vi "rdb_json_error.vi"(7 "message":string, 8 "error in (no error)":errorcluster, 10 "offset (0)":i32, 11 "json":string) -> (0 "error out":errorcluster)   [LabVIEW 2017]
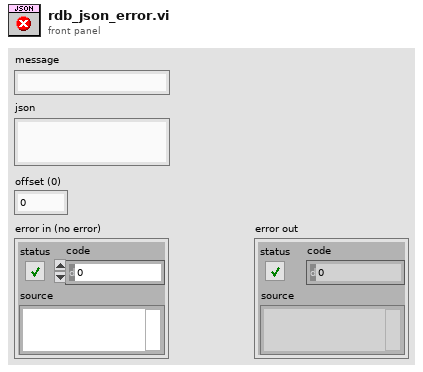
[diagram p1: front panel]
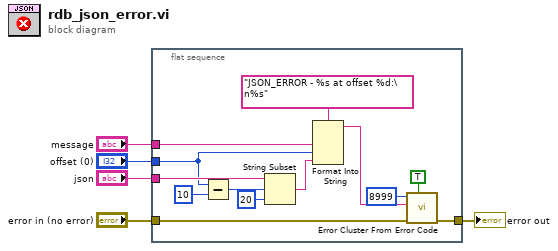
[diagram p0: block diagram]
diagram:
  n1 = flat-sequence {
    tunnel: "error in (no error)" -> [w18]
    tunnel: [w15] -> w4
    tunnel: "json" -> [w14]
    tunnel: "message" -> [w12]
    tunnel: "offset (0)" -> [w11]
    frame #0 {
      n2 = Subtract(x=w11, y=10) -> (x-y=w9:i32)
      n3 = String Subset(string=w14, offset (0)=w9, length (rest)=20 ("length (rest)")) -> (substring=w7:string)
      n4 = Format Into String(format string="JSON_ERROR - %s at offset %d:\n%s", w12, w11, w7) -> (resulting string=w6:string)  [unwired: 2 in, 1 out]
      n5 = call <vilib>:"Error Cluster From Error Code.vi"("show call chain? (False)"=TRUE, "error in (no error)"=w18, "error message (\"\")"=w6, "error code (0)"=8999) -> ("error out"=w15:errorcluster)  [unwired: 5 in]
    }
  }
  "error out" <- w4
